vi "CANRead.vi"(0 "CAN Signal":T1={"timestamp high"=0, "timestamp low"=0, "identifier"=0, "type"=enum."Data Frame", "info A"=0, "info B"=0, "data length"=0, "data"=[0, 0, 0, 0, 0, 0, 0, 0]} {"identifier" format="%x"; "timestamp high" format="%08x"; "timestamp low" format="%08x"; "data" format="%.0x"}) -> (1 "8Bytes_Received":u8[](array[numeric]), 2 "ID_Received":u32)   [LabVIEW 2013]
uses:
  <vilib>/LabVIEW Targets/FPGA/RIO/nicrio_985x_controls.llb/CAN_IO_Frame Cluster.ctl
  <vilib>/LabVIEW Targets/FPGA/RIO/nicrio_985x_controls.llb/CAN_IO_Frame Type.ctl
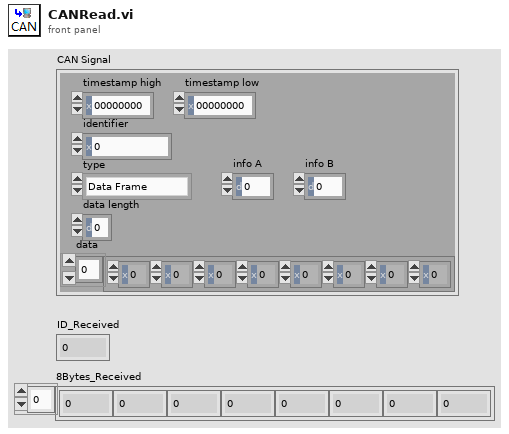
[diagram p1: front panel]
types:
  T1 = typedef "CAN_IO_Frame Cluster.ctl" = cluster{"timestamp high":u32, "timestamp low":u32, "identifier":u32, "type":T2, "info A":u8, "info B":u8, "data length":u8, "data":u8[]}
  T2 = typedef "CAN_IO_Frame Type.ctl" = enum8{"Data Frame", "Remote Frame", "(reserved)", "(reserved) ", "(reserved)  ", "(reserved)   ", "Bus Error", "Transceiver Fault"}
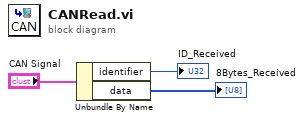
[diagram p0: block diagram]
diagram:
  n1 = Unbundle By Name("CAN Signal") -> ("identifier"=→"ID_Received":u32, "data"=→"8Bytes_Received":u8[])
